vi "background worker.vi"(8 "results reporter":refnum<class "results reporter.lvclass">, 9 "execution system":T1=enum."standard", 10 "thread pool":refnum<class "thread pool.lvclass">, 11 "connection client in":refnum<class "connection client.lvclass">) -> ()   [LabVIEW 2015, in "connection client.lvclass"]
uses:
  connection client.lvclass
  taskpool/dispatcher/thread pool.lvclass
  taskpool/dispatcher/execution system.ctl
  taskpool/results reporter/results reporter.lvclass
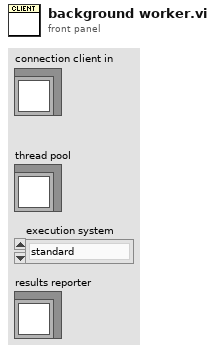
[diagram p1: front panel]
types:
  T1 = typedef "thread pool.lvclass/execution system.ctl" = enum32{"user interface", "standard", "instrument i/o", "data acquisition", "other 1", "other 2"}
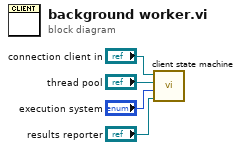
[diagram p0: block diagram]
diagram:
  n1 = call "client state machine.vi"("results reporter"="results reporter", "execution system"="execution system", "thread pool"="thread pool", "connection client in"="connection client in") -> ()  [unwired: 8 in]
